vi "CreateWaveform.vi"(8 "Simulation?":bool, 10 "Buffer Output Data":T4, 11 "Mode Estimator Processing Settings in":T1={"Low-Pass Filter Order"=5, "Downsampling Ratio"=10.0, "LPF Cut-off Frequency [Hz]"=2.5, "Sampling Frequency (Hz)"=50.0, "Parcel Length"=30000, "Detrend Cut-off Frequency (Hz)"=0.05, "AR Order"=25, "MA Order "=10, "Lower Frequency [Hz]"=0.08, "Upper Frequency [Hz]"=2.0, "Upper Damping [%]"=20.0, "Lower Damping [%]"=0.0, "Std Threshold"=1.35, "Length of Spectra [s]"=12.0, "Refresh Rate [s]"=0, "Number of critical modes"=1}) -> (1 "Mode Est Waveform":waveform(dbl), 3 "Mode Estimator Processing Settings out":T1={"Low-Pass Filter Order"=5, "Downsampling Ratio"=10.0, "LPF Cut-off Frequency [Hz]"=2.5, "Sampling Frequency (Hz)"=50.0, "Parcel Length"=30000, "Detrend Cut-off Frequency (Hz)"=0.05, "AR Order"=25, "MA Order "=10, "Lower Frequency [Hz]"=0.08, "Upper Frequency [Hz]"=2.0, "Upper Damping [%]"=20.0, "Lower Damping [%]"=0.0, "Std Threshold"=1.35, "Length of Spectra [s]"=12.0, "Refresh Rate [s]"=0, "Number of critical modes"=1})   [LabVIEW 2017]
uses:
  support/libs/PMU Buffer/Buffer DATA OUT ordered.ctl
  Mode Est Processing Settings.ctl
  <vilib>/imath/engines/lvmath2/RunTimeEngine/Managers/WorkSpace/UID Generator.vi
  <vilib>/imath/engines/lvmath/Plug In/_Char/NIMS_CH_String to Character Array.vi
  <vilib>/imath/engines/lvmath/Plug In/_Char/NIMS_CH_Character RV to String.vi
  <vilib>/imath/engines/lvmath2/RunTimeEngine/BuiltInFunctions/fread_csv/NIMS_fread_csv(Str,I32,I32).vi
  <vilib>/imath/engines/lvmath2/RunTimeEngine/RunTimeType/NIMS_RunTimeType_From StrictType (excl LVString).vi
  <instcachedir>/0/NIMS_RunTimeType_From StrictType (excl LVString)_DC56D72BB6B948F98D63F1A957D87C42.lvgen/NIMS_RunTimeType_From StrictType (excl LVString)_DC56D72BB6B948F98D63F1A957D87C42_000.vi
  <vilib>/imath/engines/lvmath2/RunTimeEngine/ErrorHandling/NIMS_Error From Error Code.vi
  <vilib>/imath/engines/lvmath2/RunTimeEngine/LocalVariableDefStatement/MC_LocalVariableDefStatement_Display.vi
  <vilib>/imath/engines/lvmath2/RunTimeEngine/Managers/SymbolTable/Clear UID.vi
  <vilib>/imath/engines/lvmath2/RunTimeEngine/NodeEndStatement/NIMS_NodeEndStatement_Output.vi
  <instcachedir>/0/NIMS_NodeEndStatement_Output_53EC0D466D134D7ABD903AC30B43404B.lvgen/NIMS_NodeEndStatement_Output_53EC0D466D134D7ABD903AC30B43404B_003.vi
  <vilib>/imath/engines/lvmath2/RunTimeEngine/ErrorHandling/NIMS_Finalize Error.vi
  <vilib>/imath/engines/lvmath2/RunTimeEngine/BuiltInFunctions/zpk_to_tf/NIMS_zpk_to_tf.vi
  <instcachedir>/0/NIMS_NodeEndStatement_Output_53EC0D466D134D7ABD903AC30B43404B.lvgen/NIMS_NodeEndStatement_Output_53EC0D466D134D7ABD903AC30B43404B_005.vi
  <vilib>/addons/Control Design/_Model Construction/Model Creation.llb/Model Creation SubVI/cd_Create Transfer Function Model.vi
  <vilib>/addons/Control Design/_Model Construction/Model Information.llb/Model Information SubVIs/cd_Set Names To TF Model.vi
  <vilib>/addons/Control Design/_Dynamic Analysis/Dynamic Analysis.llb/Dynamic Analysis subVI/cd_Damping Ratio and Natural Frequency (Transfer Function).vi
  <vilib>/addons/Control Design/_Utility/Model Viewer.llb/Model Viewer SubVI/cd_Draw Transfer Function Equation (TF).vi
  <vilib>/addons/Control Design/_Time Response Analysis/Time Response.llb/Time Response subVI/cd_Linear Simulation (Transfer Function).vi
  <vilib>/Analysis/NI_AALPro.lvlib
  <vilib>/Analysis/NI_AALBase.lvlib
  <vilib>/addons/Control Design/_Time Response Analysis/NI_CD_Time Response.lvlib
  <vilib>/addons/Control Design/_Dynamic Analysis/NI_CD_Dynamic Analysis.lvlib
  <vilib>/addons/Control Design/_Model Construction/NI_LinSys_Model Creation.lvlib
  <vilib>/addons/Control Design/_Model Construction/NI_LinSys_Model Information.lvlib
  <vilib>/addons/Control Design/_Utility/NI_CD_Model Viewer.lvlib
  <vilib>/imath/engines/lvmath2/RunTimeEngine/Managers/SymbolTable/NIMS_WorkSpace.lvlib
  support/libs/PMU Buffer/PMU data buffer.lvlib
panel:
  in  "Input Poles":cdb[](array[numeric])
  in  "Input Zeros":cdb[](array[numeric])
  in  "CSV File Input (Coefficients)":string
  out "Input Transfer Function":picture
  in  "Input Frequency (Hz)":dbl
  in  "Input Damping Ratio (%)":dbl
  in  "Simulation Method":T2(ring)
  in  "Signal Selection":T3(radio)=enum."Analog"
  out "Natural Frequencies":dbl[](array[numeric]) format="%.2f"
  out "Damping Ratios (%)":dbl[](array[numeric]) format="%.2f"
  out "Poles":cdb[](array[numeric]) format="%.2f"
  out "Simulation":bool
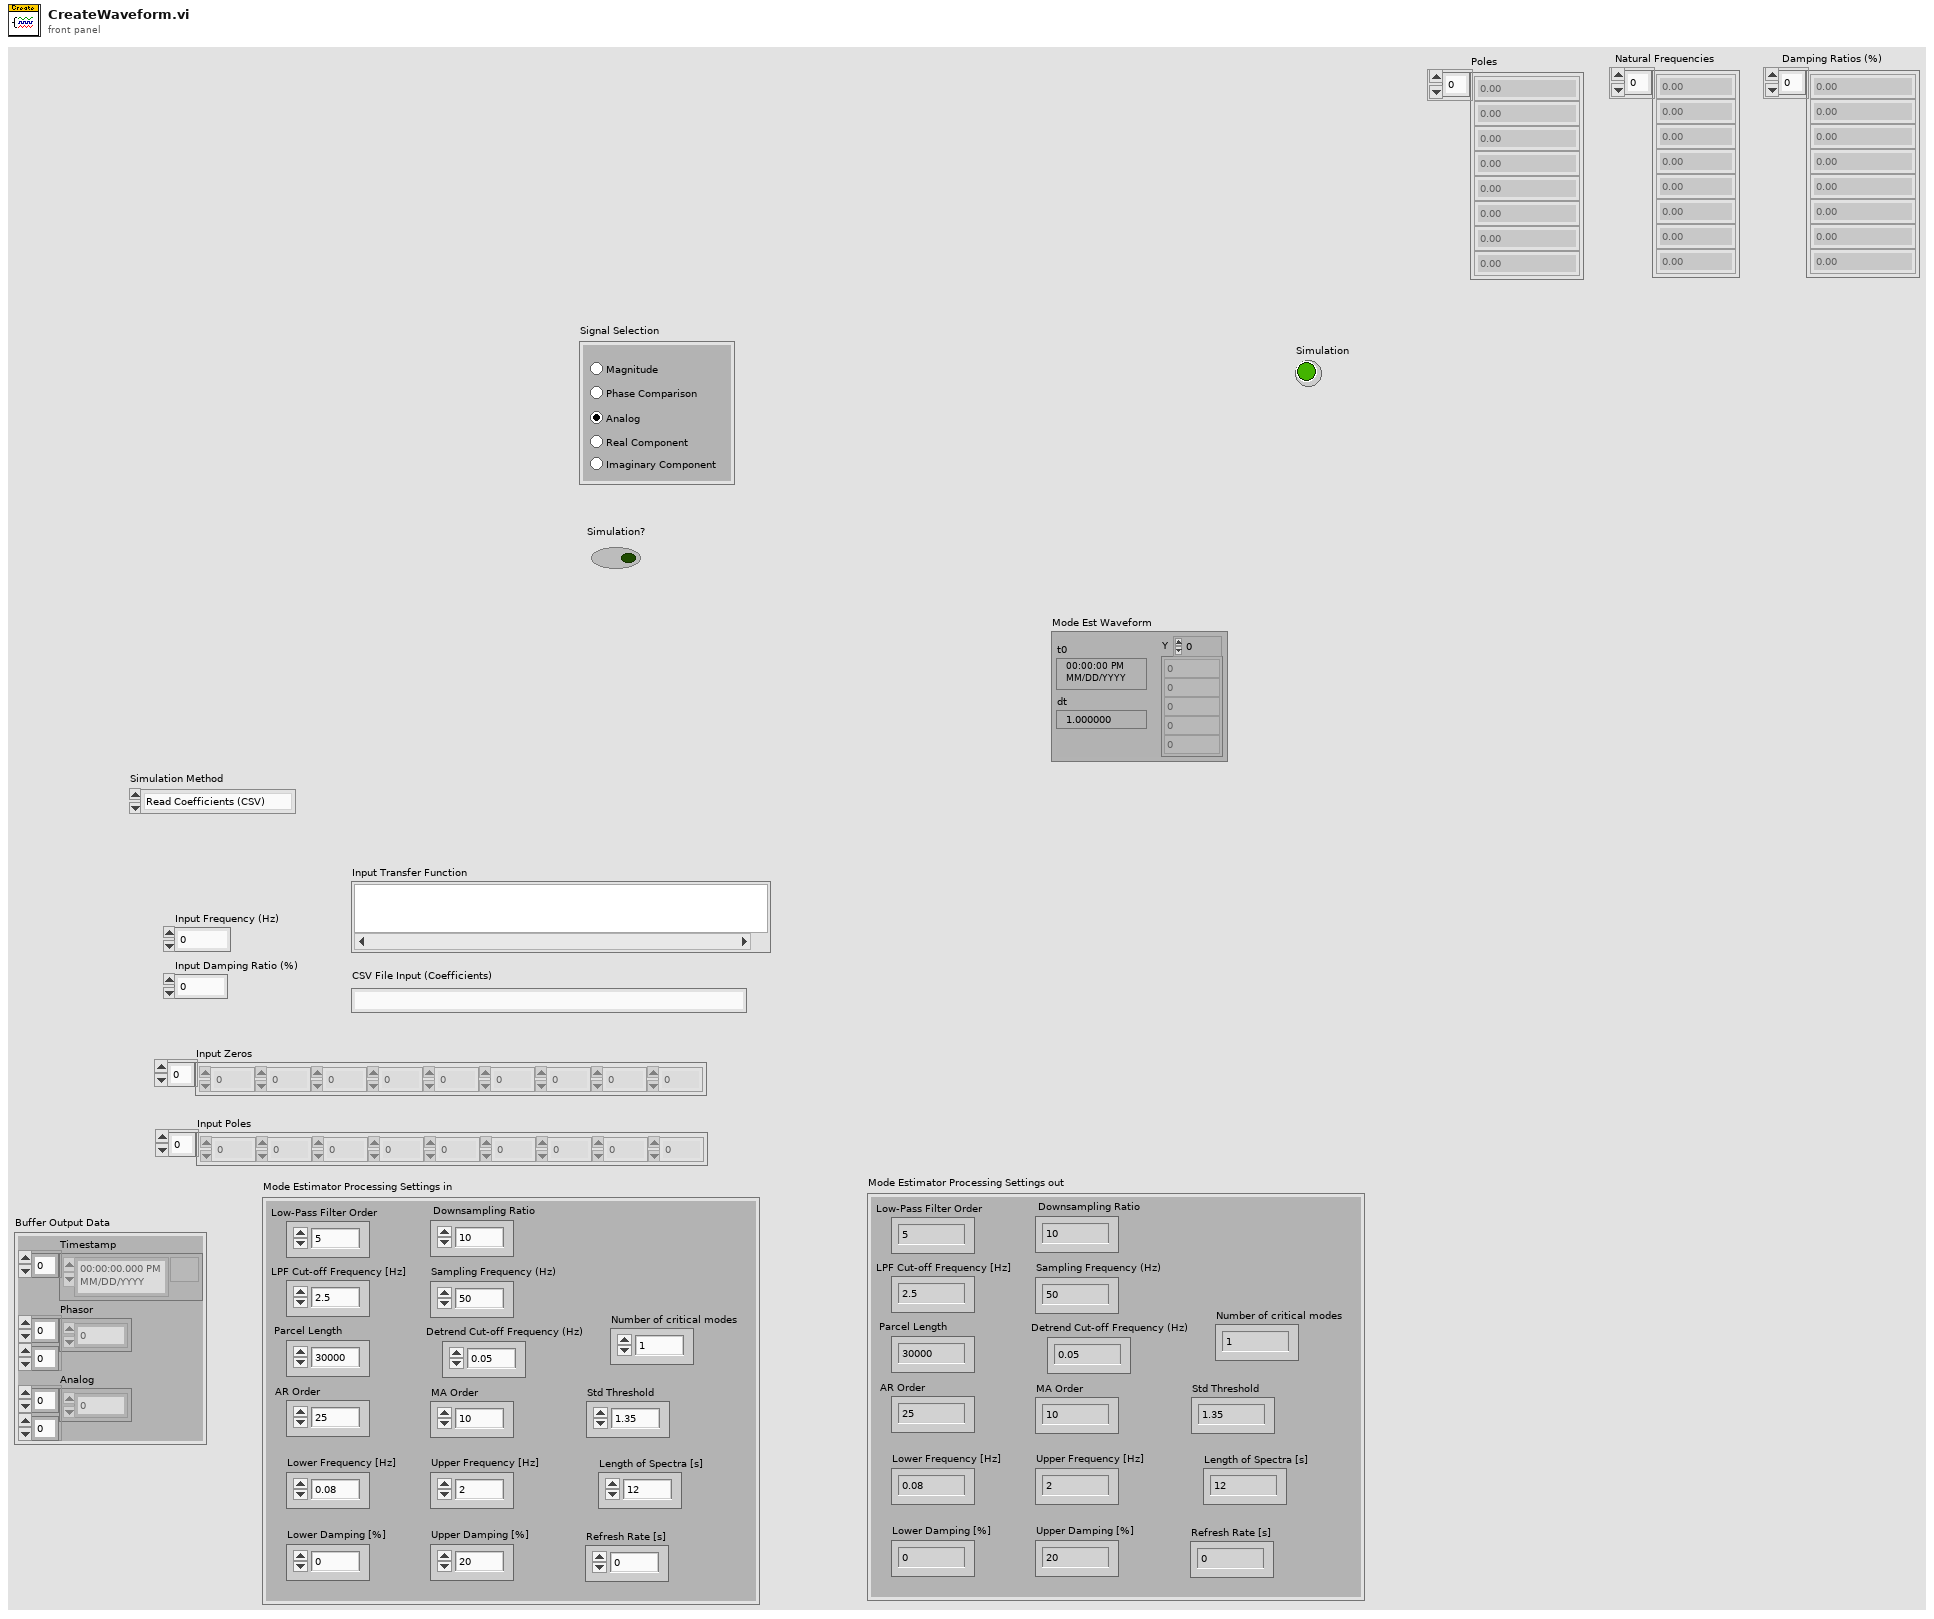
[diagram p1: front panel]
types:
  T1 = typedef "Mode Est Processing Settings.ctl" = cluster{"Low-Pass Filter Order":i32, "Downsampling Ratio":dbl, "LPF Cut-off Frequency [Hz]":dbl, "Sampling Frequency (Hz)":dbl, "Parcel Length":i32, "Detrend Cut-off Frequency (Hz)":dbl, "AR Order":i32, "MA Order ":i32, "Lower Frequency [Hz]":dbl, "Upper Frequency [Hz]":dbl, "Upper Damping [%]":dbl, "Lower Damping [%]":dbl, "Std Threshold":dbl, "Length of Spectra [s]":dbl, "Refresh Rate [s]":i32, "Number of critical modes":i32}
  T2 = enum16{"Read Coefficients (CSV)", "Use Input Frequency/D.R.", "Use Input Poles/Zeroes"}
  T3 = enum32{"Mag", "Phase Comparison", "Analog", "Real Component", "Imaginary Component"}
  T4 = typedef "PMU data buffer.lvlib/Buffer DATA OUT ordered.ctl" = cluster{"Timestamp":timestamp[], "Phasor":csg[][], "Analog":sgl[][]}
  T5 = typedef "NI_LinSys_Model Typedefs.lvlib/CD Transfer Function Model (MIMO).ctl" = cluster{"properties":T6, "transfer function(s)":T7[][]}
  T6 = typedef "NI_LinSys_Model Typedefs.lvlib/CD General Elements.ctl" = cluster{"Model name":string, "Input names":string[], "Output names":string[], "Input Delays":dbl[], "Output Delays":dbl[], "Sampling Time":dbl, "Notes":string}
  T7 = typedef "NI_LinSys_Model Typedefs.lvlib/CD Transfer Function Model (SISO).ctl" = cluster{"Numerator":dbl[], "Denominator":dbl[], "delay":dbl}
  T8 = typedef "NI_LinSys_Data Typedefs.lvlib/CD MIMO Time Response Data.ctl" = cluster{"Time":dbl[], "Outputs Data":dbl[][][], "States Data":dbl[][][], "plot type":T9}
  T9 = typedef "NI_LinSys_Data Typedefs.lvlib/CD Plot Types Enum.ctl" = enum16{"bode-magnitude", "bode-phase", "nichols", "nyquist", "singular values", "step", "impulse", "initial", "simulation", "nyquist with separation"}
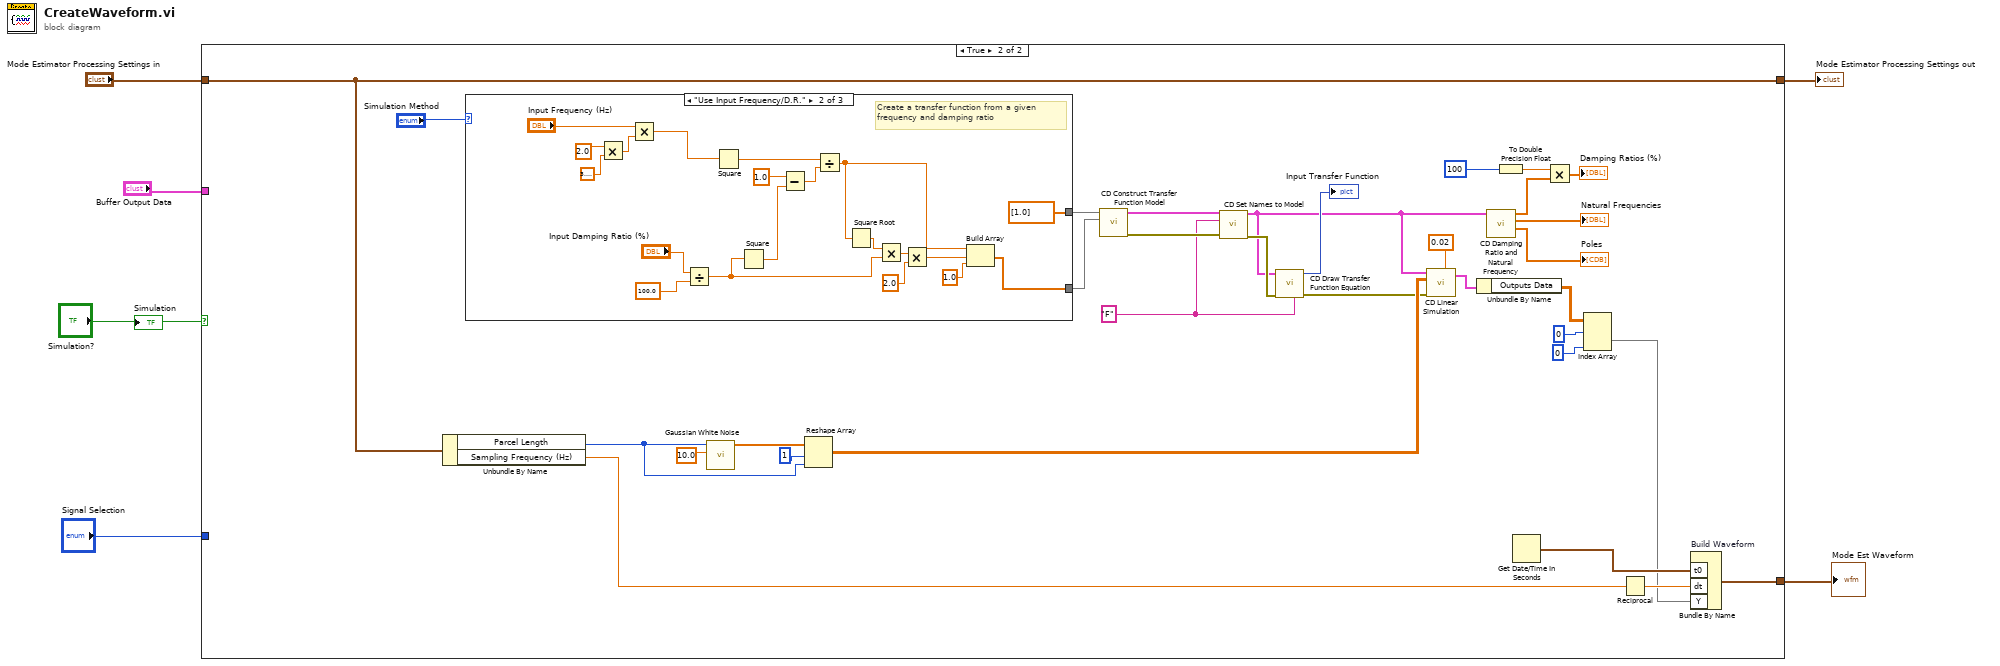
[diagram p0: block diagram]
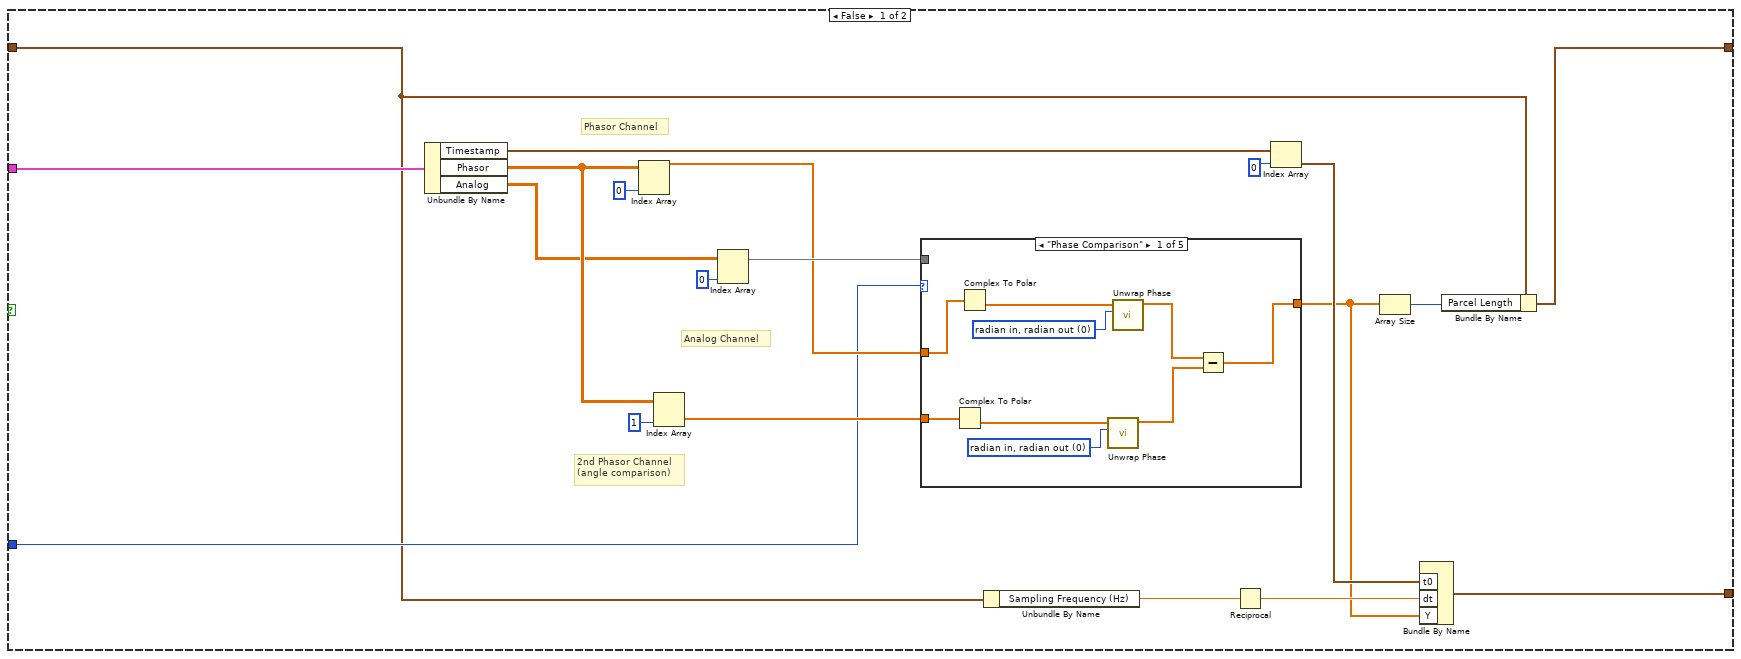
[diagram p2: hidden frame]
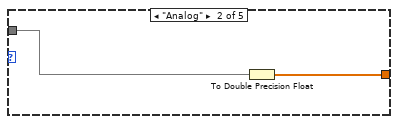
[diagram p3: hidden frame]
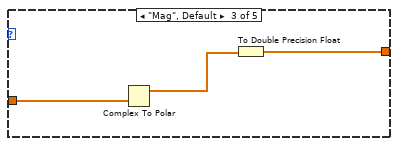
[diagram p4: hidden frame]
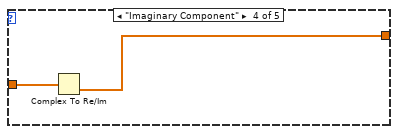
[diagram p5: hidden frame]
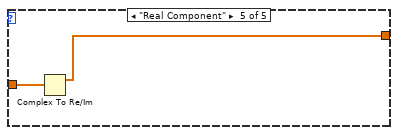
[diagram p6: hidden frame]
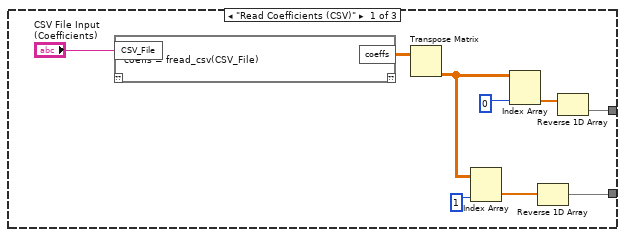
[diagram p7: hidden frame]
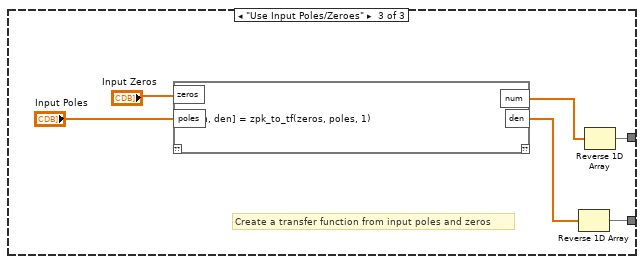
[diagram p8: hidden frame]
diagram:
  n1 = case shown="True" "Simulation?" {
    tunnel: "Buffer Output Data" -> [w15 _]
    tunnel: [w11 w48] -> w4
    tunnel: "Signal Selection" -> [w10 _]
    tunnel: "Mode Estimator Processing Settings in" -> [w9 w45]
    tunnel: [w7 w45] -> w1
    frame False {
      # "2nd Phasor Channel\n(angle comparison)"
      # "Analog Channel"
      # "Phasor Channel"
      n2 = Unbundle By Name(w15) -> ("Timestamp"=w14:timestamp[], "Phasor"=w13:csg[][], "Analog"=w12:sgl[][])
      n3 = Index Array "Index Array"(array=w13, index (col)=0 ("disabled index (col)")) -> (element=w21:csg[])  [unwired: 1 in]
      n4 = Index Array "Index Array"(array=w13, index (col)=1 ("disabled index (col)")) -> (element=w20:csg[])  [unwired: 1 in]
      n5 = Index Array "Index Array"(array=w12, index (col)=0 ("disabled index (col)")) -> (element=w22:sgl[])  [unwired: 1 in]
      n6 = case shown="\"Phase Comparison\"" w10 {
        tunnel: [w27 w37 w39 w41 w43] -> w19
        tunnel: w21 -> [w35 _ w40 w42 w44]
        tunnel: w22 -> [_ w36 _ _ _]
        tunnel: w20 -> [w30 _ _ _ _]
        frame "Phase Comparison" {
          w31 = 0 items=["radian in, radian out", "radian in, degree out", "degree in, degree out", "degree in, radian out"] ("phase unit")
          w34 = 0 items=["radian in, radian out", "radian in, degree out", "degree in, degree out", "degree in, radian out"] ("phase unit")
          n7 = Complex To Polar(r * e^(i*theta)=w30) -> (theta=w32:sgl[])  [unwired: 1 out]
          n8 = Complex To Polar(r * e^(i*theta)=w35) -> (theta=w33:sgl[])  [unwired: 1 out]
          n9 = call <vilib>:"Unwrap Phase.vi"("phase unit"=w31, "Phase"=w32) -> ("Unwrapped Phase"=w28:dbl[])  [unwired: 8 in, 1 out]
          n10 = call <vilib>:"Unwrap Phase.vi"("phase unit"=w34, "Phase"=w33) -> ("Unwrapped Phase"=w29:dbl[])  [unwired: 8 in, 1 out]
          n11 = Subtract(x=w29, y=w28) -> (x-y=w27:dbl[])
        }
        frame "Analog" {
          n12 = To Double Precision Float(number=w36) -> (double precision float=w37:dbl[])
        }
        frame "Mag", Default {
          n13 = Complex To Polar(r * e^(i*theta)=w40) -> (r=w38:sgl[])  [unwired: 1 out]
          n14 = To Double Precision Float(number=w38) -> (double precision float=w39:dbl[])
        }
        frame "Imaginary Component" {
          n15 = Complex To Re/Im(x + iy=w42) -> (y=w41:sgl[])  [unwired: 1 out]
        }
        frame "Real Component" {
          n16 = Complex To Re/Im(x + iy=w44) -> (x=w43:sgl[])  [unwired: 1 out]
        }
      }
      n17 = Unbundle By Name(w9) -> ("Sampling Frequency (Hz)"=w8:dbl)
      n18 = Reciprocal(x=w8) -> (1/x=w26:dbl)
      n19 = Index Array "Index Array"(array=w14, index=0) -> (element=w24:timestamp)
      n20 = Array Size(array=w19) -> (size(s)=w23:i32)
      n21 = Bundle By Name("t0"=w24, "dt"=w26, "Y"=w19) -> (w11:waveform(dbl))  [unwired: 1 in]
      n22 = Bundle By Name(cluster=w9, "Parcel Length"=w23) -> (w7:T1)
    }
    frame True {
      w56 = "F"
      n23 = Unbundle By Name(w45) -> ("Parcel Length"=w47:i32, "Sampling Frequency (Hz)"=w46:dbl)
      n24 = case shown="\"Use Input Frequency/D.R.\"" "Simulation Method" {
        tunnel: [w79 dbl[] [1.0] ("Array") w153] -> w54
        tunnel: [w77 w146 w155] -> w53
        frame "Read Coefficients (CSV)" {
          n25 = mathscript code="coeffs = fread_csv(CSV_File)"("CSV_File"="CSV File Input (Coefficients)") -> ("coeffs"=w82:cdb[][])  [unwired: 1 in, 1 out]
          n26 = Transpose Matrix(1:w82) -> (0:w81:cdb[][])
          n27 = Index Array "Index Array"(array=w81, index (col)=1 ("disabled index (col)")) -> (element=w78:cdb[])  [unwired: 1 in]
          n28 = Index Array "Index Array"(array=w81, index (col)=0 ("disabled index (col)")) -> (element=w80:cdb[])  [unwired: 1 in]
          n29 = Reverse 1D Array(array=w78) -> (reversed array=w77:cdb[])
          n30 = Reverse 1D Array(array=w80) -> (reversed array=w79:cdb[])
        }
        frame "Use Input Frequency/D.R." {
          # "Create a transfer function from a given\nfrequency and damping ratio"
          n31 = Multiply(x=2.0 ("y"), y=3.141592653589793) -> (x*y=w148:dbl)
          n32 = Multiply(x="Input Frequency (Hz)", y=w148) -> (x*y=w144:dbl)
          n33 = Divide(x="Input Damping Ratio (%)", y=100.0) -> (x/y=w134:dbl)
          n34 = Square(x=w144) -> (x^2=w143:dbl)
          n35 = Square(x=w134) -> (x^2=w137:dbl)
          n36 = Subtract(x=1.0 ("standard deviation"), y=w137) -> (x-y=w136:dbl)
          n37 = Divide(x=w143, y=w136) -> (x/y=w135:dbl)
          n38 = Square Root(x=w135) -> (sqrt(x)=w139:dbl)
          n39 = Multiply(x=w139, y=w134) -> (x*y=w140:dbl)
          n40 = Multiply(x=w140, y=2.0) -> (x*y=w142:dbl)
          n41 = Build Array(w135, w142, 1.0 ("standard deviation")) -> (w146:dbl[])
        }
        frame "Use Input Poles/Zeroes" {
          # "Create a transfer function from input poles and zeros"
          n42 = mathscript code="[num, den] = zpk_to_tf(zeros, poles, 1)"("zeros"="Input Zeros", "poles"="Input Poles") -> ("num"=w154:dbl[], "den"=w156:dbl[])  [unwired: 1 in, 1 out]
          n43 = Reverse 1D Array(array=w156) -> (reversed array=w155:dbl[])
          n44 = Reverse 1D Array(array=w154) -> (reversed array=w153:dbl[])
        }
      }
      n45 = call <vilib>:"Gaussian White Noise.vi"("standard deviation"=10.0, "samples"=w47) -> ("Gaussian noise pattern"=w73:dbl[])  [unwired: 8 in, 1 out]
      n46 = Reshape Array "Reshape Array"(w73, 1 ("dimension size"), w47) -> (w72:dbl[][])
      n47 = call-poly <vilib>:"CD Construct Transfer Function Model.vi"("Denominator"=w53, "Numerator"=w54) -> ("error out"=w57:errorcluster, "Transfer Function Model"=w59:T5)  [unwired: 8 in]
      n48 = call-poly <vilib>:"CD Set Names to Model.vi"("Model Name"=w56, "Transfer Function Model In"=w59, "error in (no error)"=w57) -> ("Model Out"=w49:T5, "error out"=w58:errorcluster)  [unwired: 11 in]
      n49 = call-poly <vilib>:"CD Draw Transfer Function Equation.vi"("Function Name (empty)"=w56, "error in (no error)"=w58, "Transfer Function Model"=w49) -> ("error out"=w55:errorcluster, "Equation"=→"Input Transfer Function":picture)  [unwired: 6 in, 1 out]
      n50 = call-poly <vilib>:"CD Linear Simulation.vi"("Delta t"=0.02, "error in (no error)"=w55, "Inputs"=w72, "Transfer Function Model"=w49) -> ("Simulation Data"=w71:T8)  [unwired: 5 in, 2 out]
      n51 = Unbundle By Name(w71) -> ("Outputs Data"=w69:dbl[][][])
      n52 = call-poly <vilib>:"CD Damping Ratio and Natural Frequency.vi"("Transfer Function Model"=w49) -> ("Poles"=→"Poles":cdb[], "Natural Frequencies"=→"Natural Frequencies":dbl[], "Damping Ratios"=w64:dbl[])  [unwired: 7 in, 1 out]
      n53 = To Double Precision Float(number=100 ("length")) -> (double precision float=w61:dbl)
      n54 = Get Date/Time In Seconds() -> (seconds since 1Jan1904=w75:timestamp)
      n55 = Multiply(x=w61, y=w64) -> (x*y=→"Damping Ratios (%)":dbl[])
      n56 = Index Array "Index Array"(array=w69, index (dim 0)=0 ("index"), index (dim 2)=0 ("length")) -> (element=w50:dbl[])  [unwired: 1 in]
      n57 = Reciprocal(x=w46) -> (1/x=w76:dbl)
      n58 = Bundle By Name "Build Waveform"("t0"=w75, "dt"=w76, "Y"=w50) -> (w48:waveform(dbl))  [unwired: 1 in]
    }
  }
  "Mode Est Waveform" <- w4
  "Mode Estimator Processing Settings out" <- w1
  "Simulation" <- "Simulation?"
